vi "TestHall.vi"() -> ()   [LabVIEW 2023]
uses:
  <vilib>/DAQmx/read.llb/DAQmx Read (Analog 1D DBL 1Chan NSamp).vi
  <vilib>/DAQmx/miscellaneous.llb/DAQmx Fill In Error Info.vi
panel:
  out "Numeric 2":dbl
  out "Waveform Chart 4":dynamicdata(graph)
  out "Numeric":dbl
  out "Waveform Chart 3":dbl[](graph)
  in  "?":bool
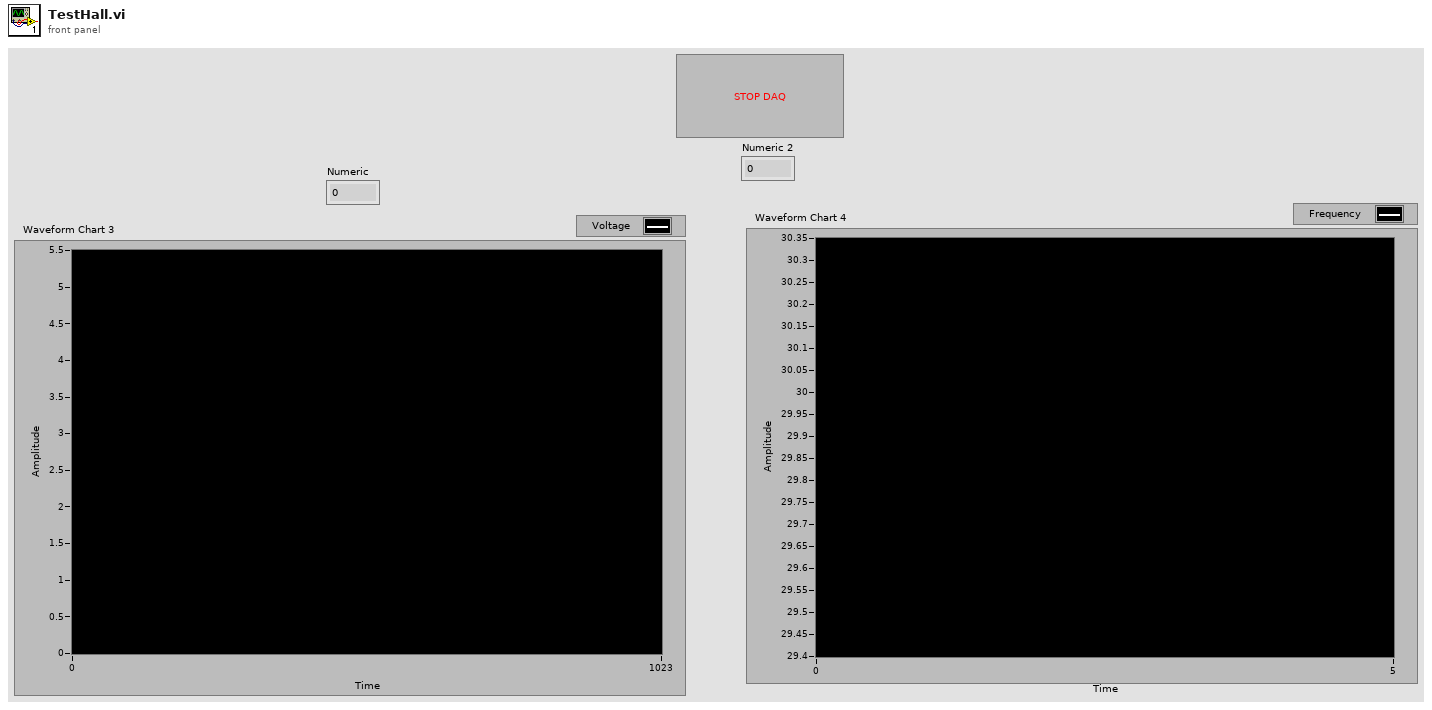
[diagram p1: front panel]
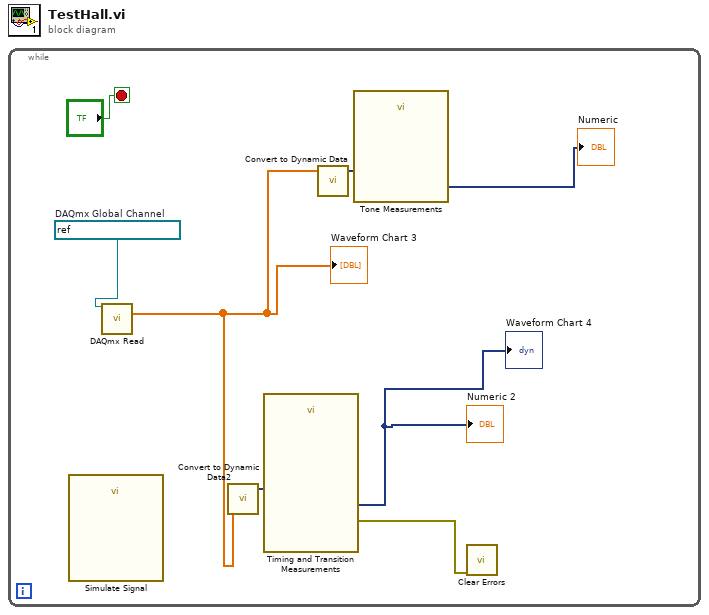
[diagram p0: block diagram]
diagram:
  n1 = while {
    stop <- "?" stop-if-true
    w7 = refnum<k21> "EfectoHallRPM"  # DAQmx Global Channel
    n2 = call "Simulate Signal"() -> ()  [unwired: 14 in, 2 out]
    n3 = call-poly <vilib>:"DAQmx Read.vi"("task/channels in"=w7) -> ("data"=w4:dbl[])  [unwired: 12 in, 2 out]
    "Waveform Chart 3" <- w4
    n4 = call "Convert to Dynamic Data2"("Array"=w4) -> ("Dynamic Data Type"=w3:dynamicdata)  [unwired: 3 in]
    n5 = call "Timing and Transition Measurements"("Signals"=w3) -> ("error out"=w2:errorcluster, "Frequency"=→"Waveform Chart 4" →"Numeric 2":dynamicdata)  [unwired: 9 in]
    n6 = call "Convert to Dynamic Data"("Array"=w4) -> ("Dynamic Data Type"=w5:dynamicdata)  [unwired: 3 in]
    n7 = call "Tone Measurements"("Signals"=w5) -> ("Frequency"=→"Numeric":dynamicdata)  [unwired: 9 in, 1 out]
    n8 = call <vilib>:"Clear Errors.vi"("error in (no error)"=w2) -> ()  [unwired: 5 in, 2 out]
  }
